vi "CREATE_VENDING MACHINE.vi"(7 "TYPE ?":bool, 8 "error in (no error)":errorcluster, 10 "PRODUCTS":T2, 11 "MONEY":T1) -> (0 "error out":errorcluster)   [LabVIEW 2019, in "DB_VENDING MACHINE.lvlib"]
doc: "En este VI se realiza el proceso para la creación de un usuario,"
uses:
  DB_VENDING MACHINE.lvlib
  Type Defs/PRODUCTS.ctl
  Type Defs/MONEY.ctl
  <vilib>/Utility/error.llb/Error Cluster From Error Code.vi
  <vilib>/ErrorRing/Error Ring.xnode
  <vilib>/addons/database/NI_Database_API.lvlib
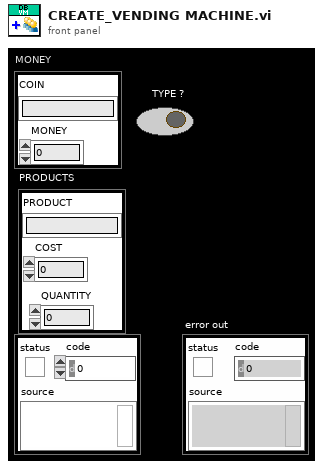
[diagram p1: front panel]
types:
  T1 = typedef "DB_VENDING MACHINE.lvlib/MONEY.ctl" = cluster{"COIN":string, "MONEY":dbl}
  T2 = typedef "DB_VENDING MACHINE.lvlib/PRODUCTS.ctl" = cluster{"PRODUCT":string, "COST":dbl, "QUANTITY":i8}
  T3 = typedef "NI_Database_API.lvlib/Conn ObjectReference.ctl" = refnum<k1>
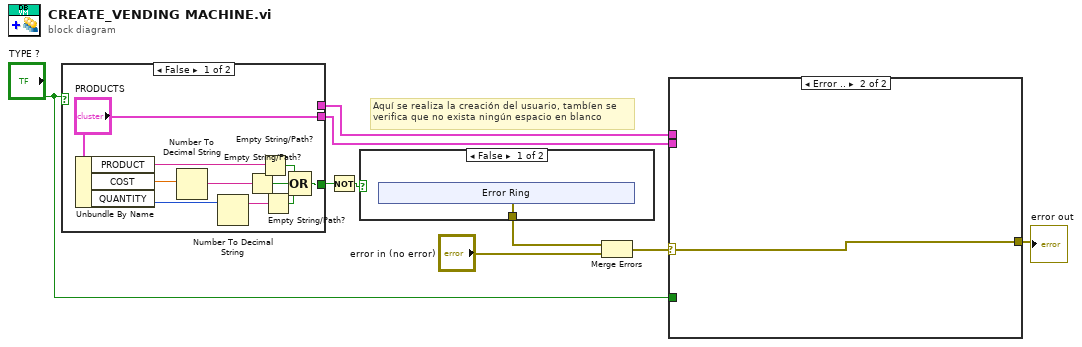
[diagram p0: block diagram]
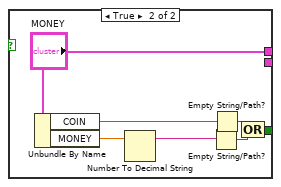
[diagram p2: hidden frame]
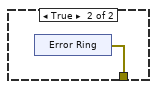
[diagram p3: hidden frame]
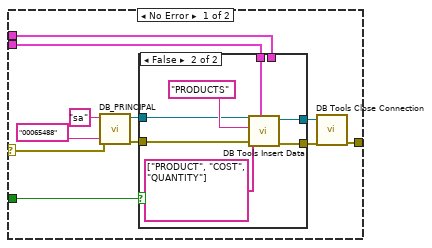
[diagram p4: hidden frame]
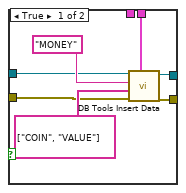
[diagram p5: hidden frame]
diagram:
  # "Aquí se realiza la creación del usuario, tambíen se\nverifica que no exista ningún espacio en blanco"
  n1 = case shown="False" "TYPE ?" {
    tunnel: ["PRODUCTS" _] -> w3
    tunnel: [_ "MONEY"] -> w1
    tunnel: [w16 w22] -> w4
    frame False {
      n2 = Unbundle By Name("PRODUCTS") -> ("PRODUCT"=w17:string, "COST"=w12:dbl, "QUANTITY"=w11:i8)
      n3 = Number To Decimal String(number=w12) -> (decimal integer string=w13:string)  [unwired: 1 in]
      n4 = Number To Decimal String(number=w11) -> (decimal integer string=w10:string)  [unwired: 1 in]
      n5 = Empty String/Path?(string/path=w13) -> (empty?=w18:bool)
      n6 = Empty String/Path?(string/path=w17) -> (empty?=w19:bool)
      n7 = Empty String/Path?(string/path=w10) -> (empty?=w14:bool)
      n8 = Compound Arithmetic op=OR(w19, w18, w14) -> (w16:bool)
    }
    frame True {
      n9 = Unbundle By Name("MONEY") -> ("COIN"=w23:string, "MONEY"=w24:dbl)
      n10 = Number To Decimal String(number=w24) -> (decimal integer string=w20:string)  [unwired: 1 in]
      n11 = Empty String/Path?(string/path=w20) -> (empty?=w25:bool)
      n12 = Empty String/Path?(string/path=w23) -> (empty?=w26:bool)
      n13 = Compound Arithmetic op=OR(w26, w25) -> (w22:bool)
    }
  }
  n14 = Not(x=w4) -> (.not. x?=w6:bool)
  n15 = case shown="False" w6 {
    tunnel: [w27 w32] -> w5
    frame False {
      n16 = xnode "Error Ring"() -> ("error out"=w27:errorcluster)
    }
    frame True {
      n17 = xnode "Error Ring"() -> ("error out"=w32:errorcluster)
    }
  }
  n18 = Merge Errors(w5, "error in (no error)") -> (w8:errorcluster)
  n19 = case shown="Error .." w8 {
    selector: w8 -> [w41 w59]
    tunnel: w3 -> [w40 _]
    tunnel: [w42 w59] -> w9
    tunnel: "TYPE ?" -> [w35 _]
    tunnel: w1 -> [w34 _]
    frame No Error {
      n20 = call "DB_PRINCIPAL.vi"("error in (no error)"=w41, "password"="00065488", "userID"="sa") -> ("error out"=w39:errorcluster, "connection reference"=w38:T3)  [unwired: 7 in]
      n21 = case shown="False" w35 {
        tunnel: w40 -> [_ w58]
        tunnel: w39 -> [w46 w57]
        tunnel: w38 -> [w49 w54]
        tunnel: [w45 w53] -> w37
        tunnel: [w48 w52] -> w36
        tunnel: w34 -> [w47 _]
        frame True {
          n22 = call <vilib>:"DB Tools Insert Data.vi"("data"=w47, "error in (no error)"=w46, "columns"=string[] ["COIN", "VALUE"], "table"="MONEY", "connection reference"=w49) -> ("error out"=w45:errorcluster, "connection reference out"=w48:T3)  [unwired: 5 in]
        }
        frame False {
          n23 = call <vilib>:"DB Tools Insert Data.vi"("data"=w58, "error in (no error)"=w57, "columns"=string[] ["PRODUCT", "COST", "QUANTITY"], "table"="PRODUCTS", "connection reference"=w54) -> ("error out"=w53:errorcluster, "connection reference out"=w52:T3)  [unwired: 5 in]
        }
      }
      n24 = call <vilib>:"DB Tools Close Connection.vi"("error in (no error)"=w37, "connection reference"=w36) -> ("error out"=w42:errorcluster)  [unwired: 5 in]
    }
    frame Error {
    }
  }
  "error out" <- w9
